vi "PinIdentifier.vi"() -> ()   [LabVIEW 2014]
uses:
  <vilib>/Platform/TimedLoop/XDataNode/timing_clust.ctl
  <vilib>/Platform/TimedLoop/XDataNode/nitl_modes.ctl
  <vilib>/Platform/TimedLoop/XDataNode/wakeup.ctl
  <vilib>/rvi/Emulation/niFpgaSctlEmulationGetInTimedLoop.vi
  <vilib>/rvi/Emulation/niFpgaEmulationReportErrorSimple.vi
  <vilib>/rvi/Emulation/niFpgaGetClockAttributes.vi
  <vilib>/rvi/Emulation/niFpgaCriticalErrorInLSC.vi
  <vilib>/rvi/eio/common/nirviEmuTemplateMethod_errors.vi
  <vilib>/Platform/TimedLoop/XDataNode/XDataNode.xnode
  <vilib>/eio/EIONode/EIONode.xnode
  <vilib>/Platform/TimedLoop/XDataNode/XDNodeRunTimeDep.lvlib
panel:
  in  "change int":u16=100
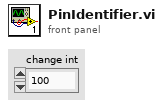
[diagram p1: front panel]
types:
  T1 = typedef "XDNodeRunTimeDep.lvlib/timing_clust.ctl" = cluster{"Expected End [f-1]":u64, "Actual End [f-1]":u64, "Finished Late? [f-1]":bool, "Expected End [i-1]":u64, "Actual End [i-1]":u64, "Finished Late? [i-1]":bool, "Expected Start [i]":u64, "Actual Start [i]":u64, "Expected Start [f]":u64, "Actual Start [f]":u64, "Source Name":string, "Structure Name":string, "Period":i64, "Deadline":i64, "Offset":i64, "Start":i64, "Priority":i32, "Timeout":i32, "Mode":T2, "Wakeup Reason":T3, "Error":errorcluster, "Source Type":string, "Secondary Source Type":string, "Global End Time":u64, "Global Start Time":u64, "Frame Duration":u64, "Iteration Duration":u64, "Assigned CPU":i32, "I/O Scan Engine Mode":u32}
  T2 = typedef "XDNodeRunTimeDep.lvlib/nitl_modes.ctl" = enum32{"No Change", "Process missed periods, maintain original phase", "Discard missed periods, maintain original phase", "Process missed periods, ignore original phase", "Discard missed periods, ignore original phase"}
  T3 = typedef "XDNodeRunTimeDep.lvlib/wakeup.ctl" = enum32{"Normal", "Aborted", "Asynchronous wakeup", "Timing source error", "Timed loop error", "Timeout"}
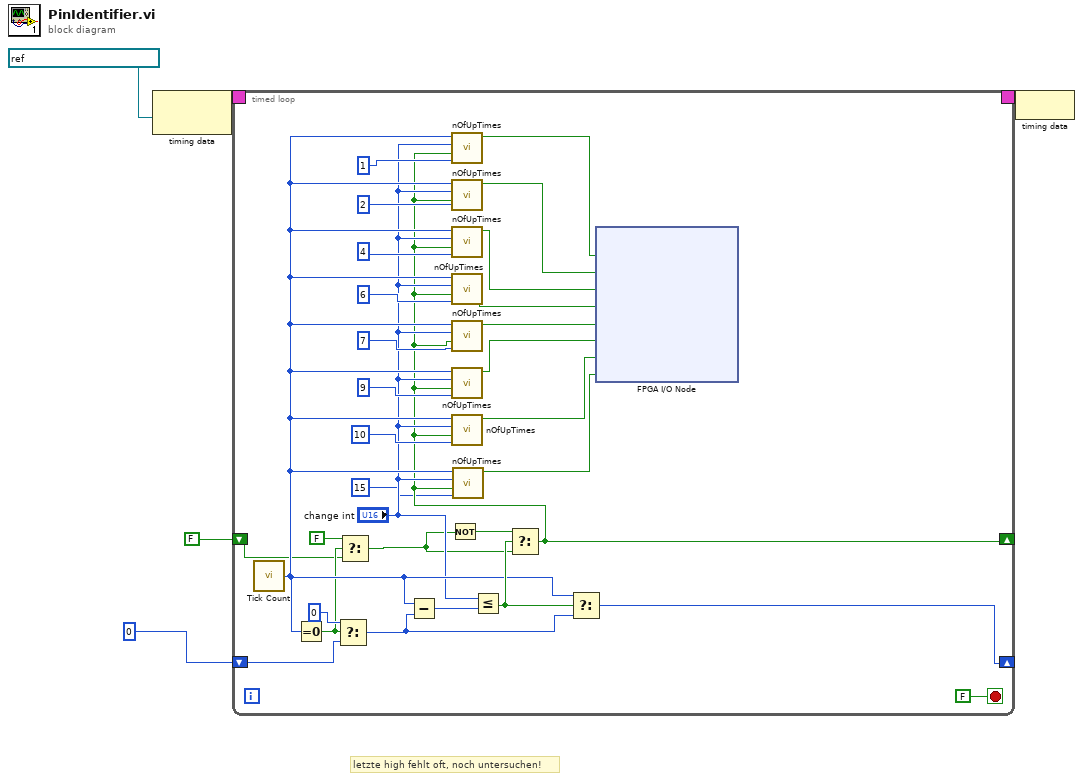
[diagram p0: block diagram]
diagram:
  # "letzte high fehlt oft, noch untersuchen!"
  n1 = node-c288(refnum<k21> "40 MHz Onboard Clock" ("Source Name")) -> (w5:T1)
  n2 = timed-loop {
    timing: w5 -> [_]
    timing-out: [_] -> w4
    shift-right: [w34] -> _
    shift-left: u16 0 ("Tick Count(Ticks)") -> [w30]
    shift-right: [w12] -> _
    shift-left: FALSE ("x < y?") -> [w8]
    stop <- FALSE stop-if-true
    n3 = call "Tick Count"() -> ("Tick Count(Ticks)"=w14:u16)
    n4 = Equal To 0?(x=w14) -> (x = 0?=w9:bool)
    n5 = Select(t=u16 0 ("Tick Count(Ticks)"), s=w9, f=w30) -> (s? t:f=w29:u16)
    n6 = Select(t=FALSE, s=w9, f=w8) -> (s? t:f=w7:bool)
    n7 = Subtract(x=w14, y=w29) -> (x-y=w35:u16)
    n8 = Not(x=w7) -> (.not. x?=w32:bool)
    n9 = Less Or Equal?(x="change int", y=w35) -> (x <= y?=w33:bool)
    n10 = Select(t=w32, s=w33, f=w7) -> (s? t:f=w12:bool)
    n11 = call "nOfUpTimes.vi"("nOfUpTimes"=u16 1, "signal"=w12, "change int"="change int", "Tick Count(Ticks)"=w14) -> ("Boolean"=w27:bool)  [unwired: 7 in]
    n12 = call "nOfUpTimes.vi"("nOfUpTimes"=u16 2, "signal"=w12, "change int"="change int", "Tick Count(Ticks)"=w14) -> ("Boolean"=w25:bool)  [unwired: 7 in]
    n13 = call "nOfUpTimes.vi"("nOfUpTimes"=u16 4, "signal"=w12, "change int"="change int", "Tick Count(Ticks)"=w14) -> ("Boolean"=w19:bool)  [unwired: 7 in]
    n14 = call "nOfUpTimes.vi"("nOfUpTimes"=u16 6, "signal"=w12, "change int"="change int", "Tick Count(Ticks)"=w14) -> ("Boolean"=w18:bool)  [unwired: 7 in]
    n15 = call "nOfUpTimes.vi"("nOfUpTimes"=u16 7, "signal"=w12, "change int"="change int", "Tick Count(Ticks)"=w14) -> ("Boolean"=w17:bool)  [unwired: 7 in]
    n16 = call "nOfUpTimes.vi"("nOfUpTimes"=u16 9, "signal"=w12, "change int"="change int", "Tick Count(Ticks)"=w14) -> ("Boolean"=w16:bool)  [unwired: 7 in]
    n17 = call "nOfUpTimes.vi"("nOfUpTimes"=u16 10, "signal"=w12, "change int"="change int", "Tick Count(Ticks)"=w14) -> ("Boolean"=w15:bool)  [unwired: 7 in]
    n18 = call "nOfUpTimes.vi"("nOfUpTimes"=u16 15, "signal"=w12, "change int"="change int", "Tick Count(Ticks)"=w14) -> ("Boolean"=w10:bool)  [unwired: 7 in]
    n19 = Select(t=w14, s=w33, f=w29) -> (s? t:f=w34:u16)
    n20 = xnode "FPGA I/O Node"("MISO"=w27, "RESET"=w25, "CLR"=w19, "LDAC"=w18, "MOSI"=w17, "SCLK"=w16, "CS"=w15, "Connector2/DIO35"=w10) -> ()  [unwired: 8 in, 8 out]
  }
  n21 = node-c288(w4) -> ()
